vi "UTIL_LevelStatus.vi"(10 "Status In in":i16, 11 "Good!Bad":bool) -> (1 "Err Num":i32, 3 "Status In out":u32)   [LabVIEW 2024]
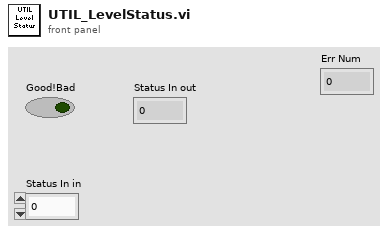
[diagram p1: front panel]
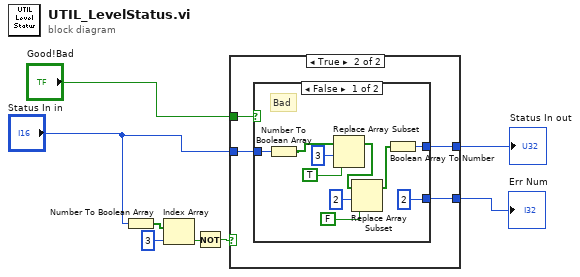
[diagram p0: block diagram]
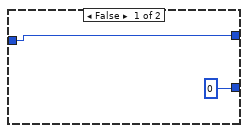
[diagram p2: hidden frame]
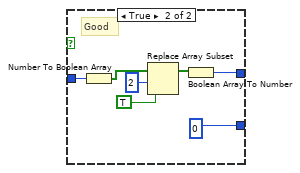
[diagram p3: hidden frame]
diagram:
  n1 = Number To Boolean Array(number="Status In in") -> (Boolean array=w2:bool[])
  n2 = Index Array(array=w2, index=3) -> (element=w4:bool)
  n3 = Not(x=w4) -> (.not. x?=w6:bool)
  n4 = case shown="True" w6 {
    tunnel: "Good!Bad" -> [_ w14]
    tunnel: [w10 w13] -> w8
    tunnel: "Status In in" -> [w10 w12]
    tunnel: [0 w11] -> w1
    frame False {
    }
    frame True {
      n5 = case shown="False" w14 {
        tunnel: w12 -> [w22 w29]
        tunnel: [w20 w26] -> w13
        tunnel: [2 0] -> w11
        frame False {
          # "Bad"
          n6 = Number To Boolean Array(number=w22) -> (Boolean array=w21:bool[])
          n7 = Replace Array Subset(array=w21, new element=TRUE ("new element/subarray"), index=3) -> (w17:bool[])
          n8 = Replace Array Subset(array=w17, new element=FALSE ("new element/subarray"), index=2) -> (w16:bool[])
          n9 = Boolean Array To Number(Boolean array=w16) -> (number=w20:u32)
        }
        frame True {
          # "Good"
          n10 = Number To Boolean Array(number=w29) -> (Boolean array=w28:bool[])
          n11 = Replace Array Subset(array=w28, new element=TRUE ("new element/subarray"), index=2) -> (w27:bool[])
          n12 = Boolean Array To Number(Boolean array=w27) -> (number=w26:u32)
        }
      }
    }
  }
  "Status In out" <- w8
  "Err Num" <- w1
